vi "题目5.vi"() -> ()   [LabVIEW 2017]
panel:
  out "恭喜":bool
  out "通过":bool
  out "警告":bool
  in  "数值":dbl
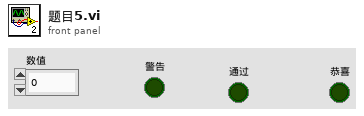
[diagram p1: front panel]
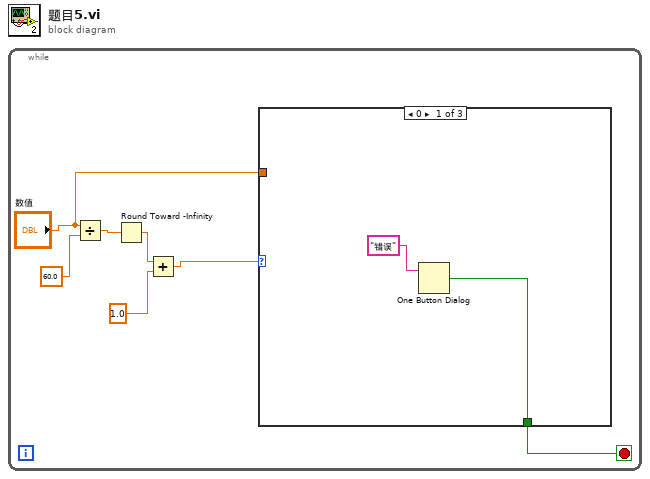
[diagram p0: block diagram]
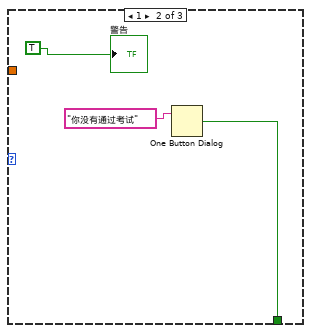
[diagram p2: hidden frame]
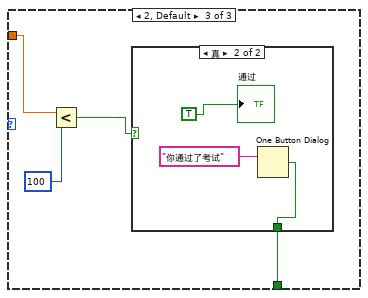
[diagram p3: hidden frame]
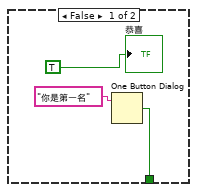
[diagram p4: hidden frame]
diagram:
  n1 = while {
    stop <- w1 stop-if-true
    n2 = Divide(x="数值", y=60.0) -> (x/y=w6:dbl)
    n3 = Round Toward -Infinity(1:w6) -> (0:w4:dbl)
    n4 = Add(x=w4, y=1.0) -> (x+y=w3:dbl)
    n5 = case shown="0" w3 {
      tunnel: "数值" -> [_ _ w16]
      tunnel: [w8 w10 w13] -> w1
      frame 0 {
        n6 = One Button Dialog(message="错误") -> (true=w8:bool)  [unwired: 1 in]
      }
      frame 1 {
        n7 = One Button Dialog(message="你没有通过考试") -> (true=w10:bool)  [unwired: 1 in]
        "警告" <- TRUE
      }
      frame 2, Default {
        n8 = Less?(x=w16, y=100) -> (x < y?=w14:bool)
        n9 = case shown="真" w14 {
          tunnel: [w17 w20] -> w13
          frame False {
            n10 = One Button Dialog(message="你是第一名") -> (true=w17:bool)  [unwired: 1 in]
            "恭喜" <- TRUE
          }
          frame True {
            n11 = One Button Dialog(message="你通过了考试") -> (true=w20:bool)  [unwired: 1 in]
            "通过" <- TRUE
          }
        }
      }
    }
  }
